vi "diagonal cross A.vi"(10 "A":T1, 11 "diagonal":dbl[](array[numeric])) -> (3 "diagonalxA":T1)   [LabVIEW 2017, in "NI_Gmath.lvlib"]
uses:
  NI_Gmath.lvlib
  RealMatrix.ctl
  NI_Matrix.lvlib
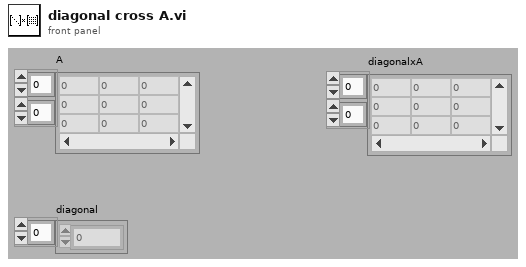
[diagram p1: front panel]
types:
  T1 = typedef "NI_Matrix.lvlib/RealMatrix.ctl" = dbl[][]
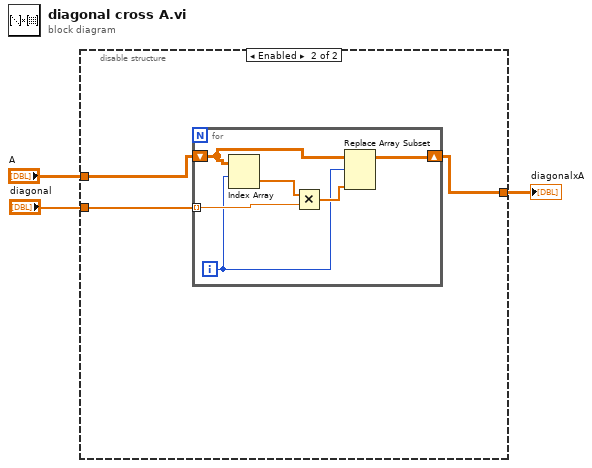
[diagram p0: block diagram]
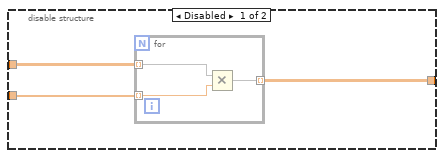
[diagram p2: hidden frame]
diagram:
  n1 = disable-structure shown="Enabled" {
    disable-tunnel: "A" -> [w6 w12]
    disable-tunnel: "diagonal" -> [w5 w11]
    disable-tunnel: [w4 w10] -> w1
    frame Disabled {
      n2 = for {
        tunnel: w6 -> [w9] mode=indexing
        tunnel: w5 -> [w8] mode=indexing
        tunnel: [w7] -> w4 mode=indexing
        n3 = Multiply(x=w9, y=w8) -> (x*y=w7:dbl[])
      }
    }
    frame Enabled {
      n4 = for {
        tunnel: w11 -> [w18] mode=indexing
        shift-right: [w14] -> w10
        shift-left: w12 -> [w17]
        i -> [w13]
        n5 = Index Array(array=w17, index (row)=w13) -> (element=w16:dbl[])  [unwired: 1 in]
        n6 = Multiply ("Multiply.vi")(x=w16, y=w18) -> (x*y=w15:dbl[])
        n7 = Replace Array Subset(array=w17, new element=w15, index (row)=w13) -> (w14:T1)  [unwired: 1 in]
      }
    }
  }
  "diagonalxA" <- w1
